vi "scope_DAQ_test.vi"() -> ()   [LabVIEW 2020]
uses:
  LeCroy Wave Series/LeCroy Wave Series.lvlib
panel:
  out "#  IR On Len":i32
  out "# IR Off len":i32
  out "Gate Trace":waveform(dbl)(graph)
  in  "Legacy Mode 2":bool
  in  "Main Tab Control":T1(tab)
  in  "Scope Trace Tabs":enum32{"Raw Trace", "Avg Traces", "IR Spectrum"}(tab)
  out "Raw Trace":waveform(dbl)(graph)
  in  "Data Channel (0: Channel 1)":u16(ring) items=["Channel 1", "Channel 2", "Channel 3", "Channel 4", "Memory 1", "Memory 2", "Memory 3", "Memory 4", "Function 1", "Function 2", "Function 3", "Function 4", "Function 5", "Function 6", "Function 7", "Function 8", "Other"]
  in  "Number of Sweeps":i32
  in  "Scope On/Off":bool
  in  "stop":bool
  out "Consumer Loop Time / ms":u32
  out "Producer Loop Time / ms":u32
  in  "ID Query? (T: Yes)":bool
  in  "Reset? (T: Yes)":bool
  in  "Auto Setup Scope":bool
  in  "Laser gate threshold":dbl
  # "Ensure that the cursors are gating the peak you are recording the spectrum on if you want a real time spectrum!"
  # "LEAVE THESE ALONE UNLESS YOU KNOW WHAT YOU ARE DOING!"
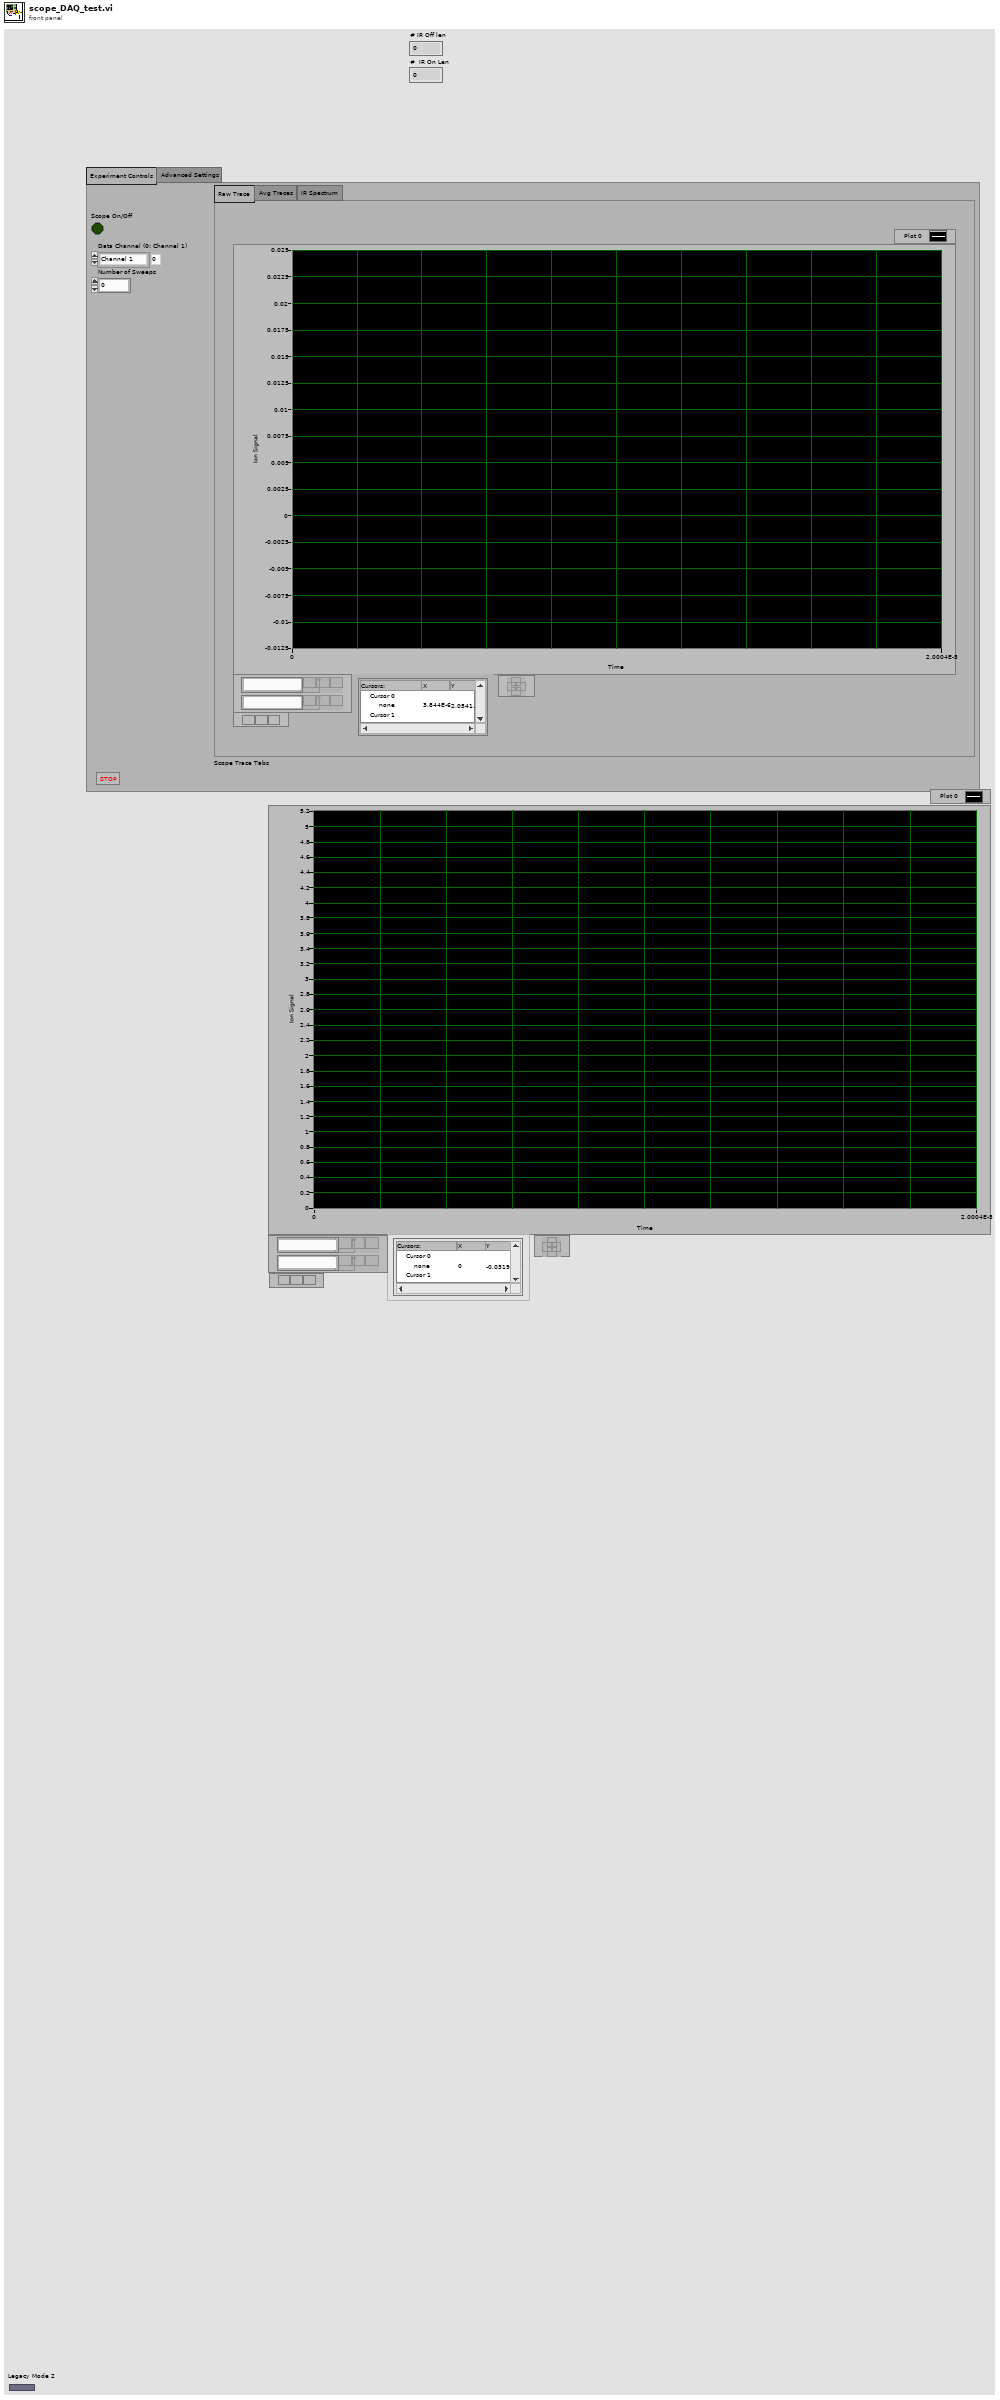
[diagram p1: front panel]
types:
  T1 = enum32{"Experiment Controls", "Advanced Settings"}
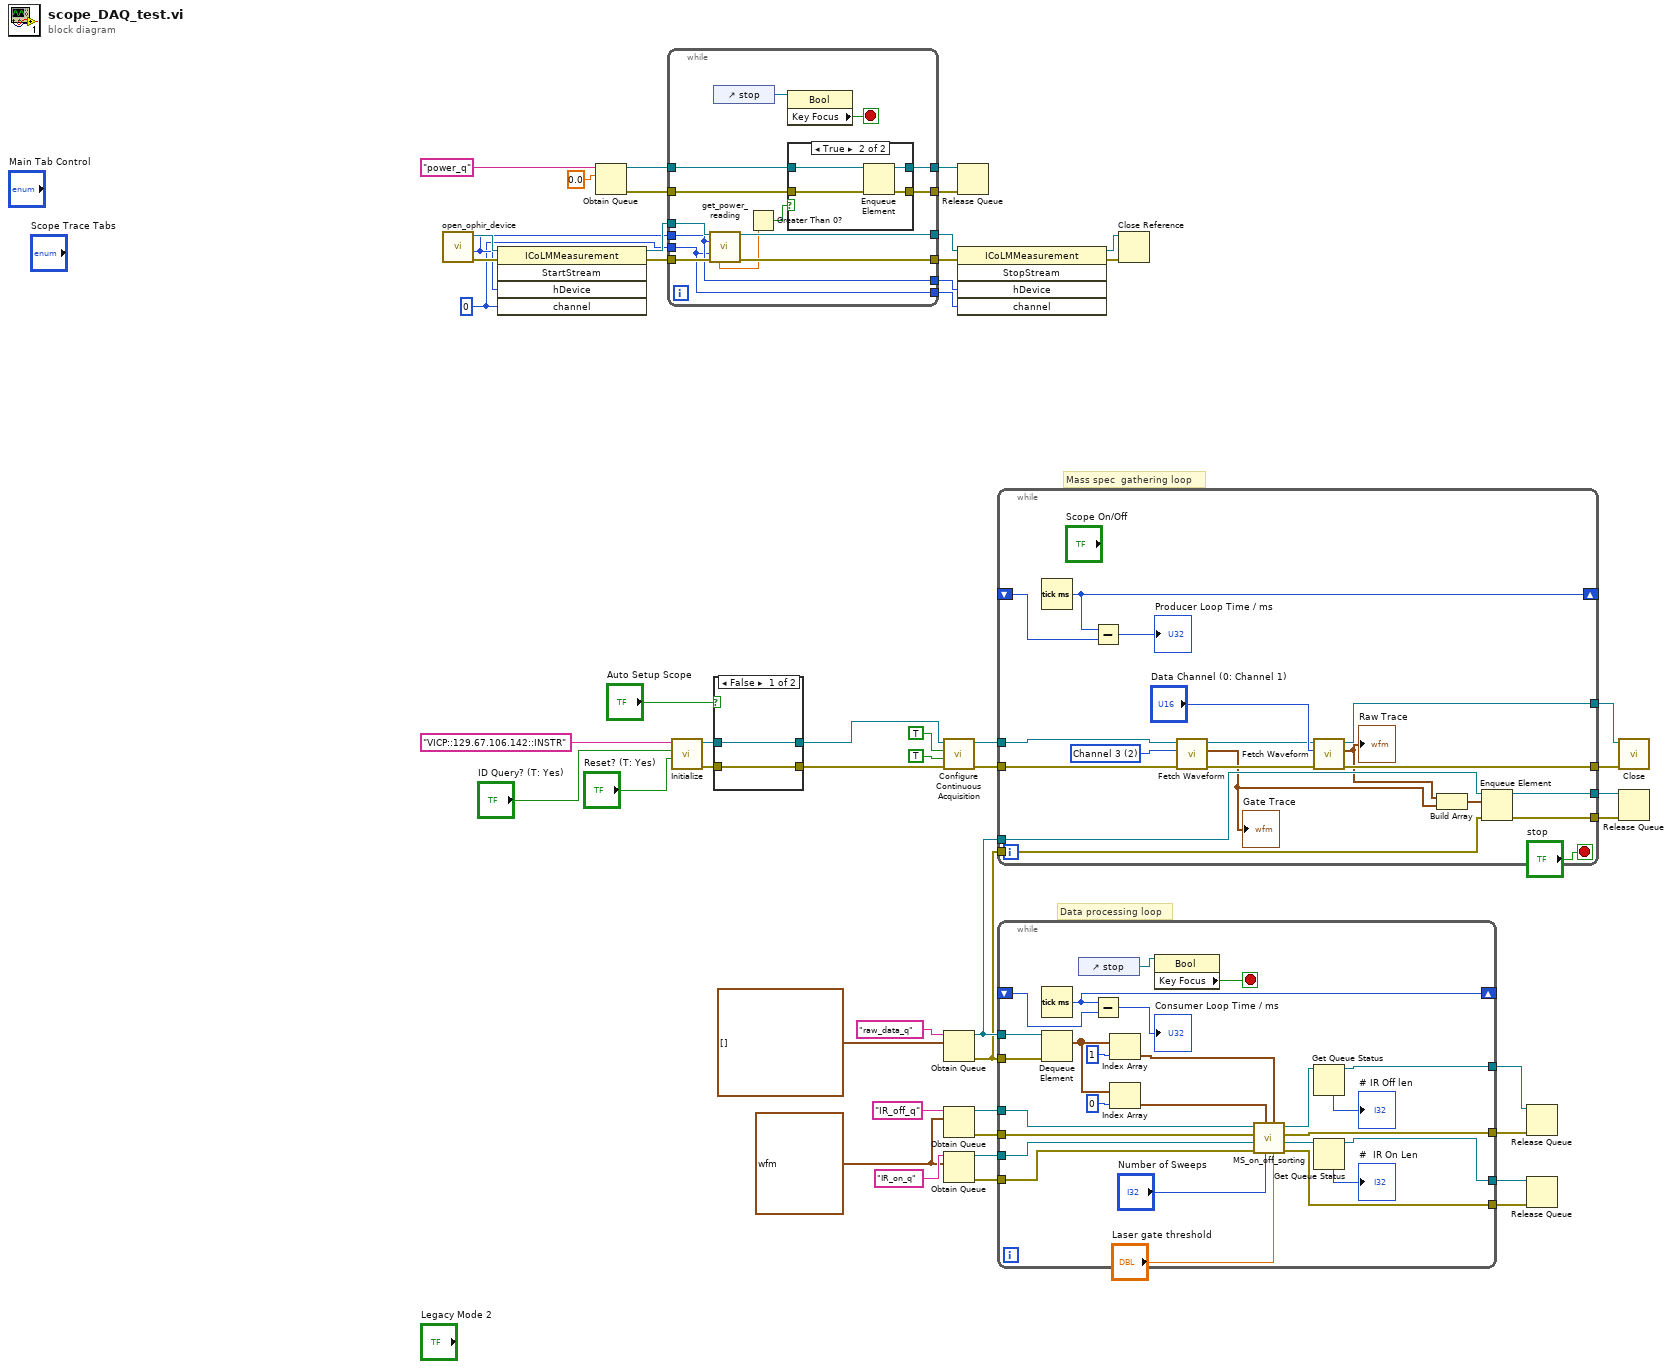
[diagram p0: block diagram]
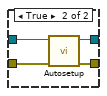
[diagram p3: hidden frame]
diagram:
  w19 = waveform(dbl) {"t0"=timestamp(0 s since 1904-01-01), "dt"=1.0, "Y"=[]} ("element")
  w27 = 0 ("channel")
  # "Data processing loop"
  # "Mass spec  gathering loop"
  n1 = call "open_ophir_device.vi"() -> ("error out"=w33:errorcluster, "hDevice"=w28:i32, "Orphir COM"=w34:refnum<k7>)  [unwired: 7 in, 2 out]
  n2 = invoke class="ICoLMMeasurement" method="StartStream"(reference=w34, error in=w33, "hDevice"=w28, "channel"=w27) -> (reference out=w30:refnum<k7>, error out=w29:errorcluster)  [unwired: 1 in, 3 out]
  n3 = Obtain Queue(name (unnamed)="power_q", element data type=0.0) -> (queue out=w1:refnum<queue>, error out=w4:errorcluster)  [unwired: 3 in, 1 out]
  n4 = while {
    tunnel: w30 -> [w63]
    tunnel: w29 -> [w62]
    tunnel: w28 -> [w59]
    tunnel: w27 -> [w58]
    tunnel: [w61] -> w26
    tunnel: [w60] -> w25
    tunnel: [w59] -> w24
    tunnel: [w58] -> w23
    tunnel: w1 -> [w57]
    tunnel: w4 -> [w56]
    tunnel: [w55] -> w3
    tunnel: [w54] -> w2
    stop <- w50 stop-if-true
    n5 = call "get_power_reading.vi"("reference in"=w63, "hDevice"=w59, "channel"=w58, "error in (no error)"=w62) -> ("reference out"=w61:refnum<k7>, "Power / J"=w52:dbl, "error out"=w60:errorcluster)  [unwired: 5 in, 4 out]
    n6 = control-ref of="stop"() -> (w51:refnum<vi>)
    n7 = Greater Than 0?(x=w52) -> (x > 0?=w53:bool)
    n8 = property class="Bool"(reference=w51) -> ("Key Focus"=w50:bool)  [unwired: 1 in, 2 out]
    n9 = case shown="True" w53 {
      tunnel: w57 -> [w65 w69]
      tunnel: w56 -> [w64 w68]
      tunnel: [w65 w67] -> w55
      tunnel: [w64 w66] -> w54
      frame False {
      }
      frame True {
        n10 = Enqueue Element(queue=w69, error in (no error)=w68) -> (queue out=w67:refnum<queue>, error out=w66:errorcluster)  [unwired: 2 in, 1 out]
      }
    }
  }
  n11 = call "Initialize.vi"("Reset? (T: Yes)"="Reset? (T: Yes)", "ID Query? (T: Yes)"="ID Query? (T: Yes)", "VISA resource name"="VICP::129.67.106.142::INSTR") -> ("error out"=w48:errorcluster, "VISA resource name out"=w49:refnum<visa-resource-name>)  [unwired: 7 in]
  n12 = case shown="False" "Auto Setup Scope" {
    tunnel: w49 -> [w71 w75]
    tunnel: w48 -> [w70 w74]
    tunnel: [w71 w73] -> w47
    tunnel: [w70 w72] -> w46
    frame False {
    }
    frame True {
      n13 = call "Autosetup.vi"("error in (no error)"=w74, "VISA resource name"=w75) -> ("error out"=w72:errorcluster, "VISA resource name out"=w73:refnum<visa-resource-name>)  [unwired: 8 in]
    }
  }
  n14 = call "Configure Continuous Acquisition.vi"("error in (no error)"=w46, "Auto Trigger Enabled (T: Normal)"=TRUE, "Continuous Acquisition Mode (T: On)"=TRUE, "VISA resource name"=w47) -> ("error out"=w42:errorcluster, "VISA resource name out"=w43:refnum<visa-resource-name>)  [unwired: 6 in]
  n15 = Obtain Queue(name (unnamed)="raw_data_q", element data type=waveform(dbl)[] [] ("appended array")) -> (queue out=w8:refnum<queue>, error out=w7:errorcluster)  [unwired: 3 in, 1 out]
  n16 = Obtain Queue(name (unnamed)="IR_off_q", element data type=w19) -> (queue out=w18:refnum<queue>, error out=w17:errorcluster)  [unwired: 3 in, 1 out]
  n17 = Obtain Queue(name (unnamed)="IR_on_q", element data type=w19) -> (queue out=w16:refnum<queue>, error out=w15:errorcluster)  [unwired: 3 in, 1 out]
  n18 = Release Queue(queue=w3, error in (no error)=w2) -> ()  [unwired: 1 in, 3 out]
  n19 = invoke class="ICoLMMeasurement" method="StopStream"(reference=w26, error in=w25, "hDevice"=w24, "channel"=w23) -> (reference out=w32:refnum<k7>, error out=w31:errorcluster)  [unwired: 1 in, 3 out]
  n20 = while {
    tunnel: w43 -> [w85]
    tunnel: w42 -> [w84]
    tunnel: [w94] -> w40
    tunnel: [w93] -> w39
    tunnel: w8 -> [w82]
    tunnel: [w80] -> w10
    tunnel: w7 -> [w81]
    tunnel: [w79] -> w9
    shift-right: [w91] -> _
    shift-left: _ -> [w92]
    stop <- "stop" stop-if-true
    w83 = u16 2 items=["Channel 1", "Channel 2", "Channel 3", "Channel 4", "Memory 1", "Memory 2", "Memory 3", "Memory 4", "Function 1", "Function 2", "Function 3", "Function 4", "Function 5", "Function 6", "Function 7", "Function 8", "Other"] ("Source (0: Channel 1)")
    n21 = Tick Count (ms)() -> (millisecond timer value=w91:u32)
    n22 = Subtract(x=w91, y=w92) -> (x-y=→"Producer Loop Time / ms":u32)
    n23 = call "Fetch Waveform.vi"("error in (no error)"=w84, "Source (0: Channel 1)"=w83, "VISA resource name"=w85) -> ("error out"=w86:errorcluster, "Waveform Graph"=w77:waveform(dbl), "VISA resource name out"=w87:refnum<visa-resource-name>)  [unwired: 6 in]
    "Gate Trace" <- w77
    n24 = call "Fetch Waveform.vi"("error in (no error)"=w86, "Source (0: Channel 1)"="Data Channel (0: Channel 1)", "VISA resource name"=w87) -> ("error out"=w93:errorcluster, "Waveform Graph"=w78:waveform(dbl), "VISA resource name out"=w94:refnum<visa-resource-name>)  [unwired: 6 in]
    "Raw Trace" <- w78
    n25 = Build Array(w78, w77) -> (w76:waveform(dbl)[])
    n26 = Enqueue Element(queue=w82, element=w76, error in (no error)=w81) -> (queue out=w80:refnum<queue>, error out=w79:errorcluster)  [unwired: 1 in, 1 out]
  }
  n27 = while {
    tunnel: w18 -> [w115]
    tunnel: w17 -> [w113]
    tunnel: w16 -> [w114]
    tunnel: w15 -> [w112]
    shift-right: [w116] -> _
    shift-left: _ -> [w117]
    tunnel: [w101] -> w14
    tunnel: [w111] -> w13
    tunnel: [w99] -> w12
    tunnel: [w110] -> w11
    tunnel: w8 -> [w96]
    tunnel: w7 -> [w95]
    stop <- w119 stop-if-true
    n28 = Tick Count (ms)() -> (millisecond timer value=w116:u32)
    n29 = Dequeue Element(queue=w96, error in (no error)=w95) -> (element=w109:waveform(dbl)[])  [unwired: 1 in, 3 out]
    n30 = control-ref of="stop"() -> (w120:refnum<vi>)
    n31 = Subtract(x=w116, y=w117) -> (x-y=→"Consumer Loop Time / ms":u32)
    n32 = Index Array(array=w109, index=1) -> (element=w106:waveform(dbl))
    n33 = Index Array(array=w109, index=0) -> (element=w105:waveform(dbl))
    n34 = property class="Bool"(reference=w120) -> ("Key Focus"=w119:bool)  [unwired: 1 in, 2 out]
    n35 = call "MS_on_off_sorting.vi"("Laser gate threshold"="Laser gate threshold", "gate_trace"=w106, "Number of sweeps"="Number of Sweeps", "data_trace"=w105, "IR_on_q_error_in"=w112, "IR_on_q_in"=w114, "IR_off_q_error_in"=w113, "IR_off_q_in"=w115) -> ("IR_on_q_error_out"=w110:errorcluster, "IR_on_q_out"=w100:refnum<queue>, "IR_off_q_error_out"=w111:errorcluster, "IR_off_q_out"=w102:refnum<queue>)
    n36 = Get Queue Status(queue=w102) -> (queue out=w101:refnum<queue>, # elements in queue=→"# IR Off len":i32)  [unwired: 2 in, 6 out]
    n37 = Get Queue Status(queue=w100) -> (queue out=w99:refnum<queue>, # elements in queue=→"#  IR On Len":i32)  [unwired: 2 in, 6 out]
  }
  n38 = Close Reference(reference=w32, error in (no error)=w31) -> ()  [unwired: 1 out]
  n39 = Release Queue(queue=w14, error in (no error)=w13) -> ()  [unwired: 1 in, 3 out]
  n40 = Release Queue(queue=w12, error in (no error)=w11) -> ()  [unwired: 1 in, 3 out]
  n41 = call "Close.vi"("error in (no error)"=w39, "VISA resource name"=w40) -> ()  [unwired: 9 in, 1 out]
  n42 = Release Queue(queue=w10, error in (no error)=w9) -> ()  [unwired: 1 in, 3 out]
